vi "test_scd_main.vi"(8 "error in":errorcluster) -> (0 "error out":errorcluster)   [LabVIEW 2023, in "horiba.test.lvlib"]
uses:
  horiba.test.lvlib
  Classes/SCD/SCD.lvclass
  <vilib>/addons/_JKI Toolkits/Caraya/classes/Test/Test.lvclass
  C:/Projects/Horiba/horiba-labview-sdk/Source/Classes/GenericDevice/GenericDevice.lvclass
  C:/Projects/Horiba/horiba-labview-sdk/Source/Classes/SCD/SCD.lvclass
panel:
  # "Connector Pane"
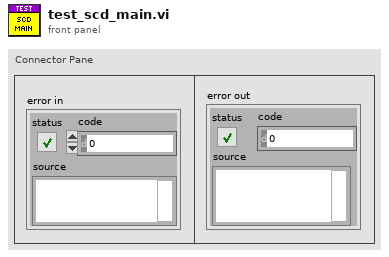
[diagram p1: front panel]
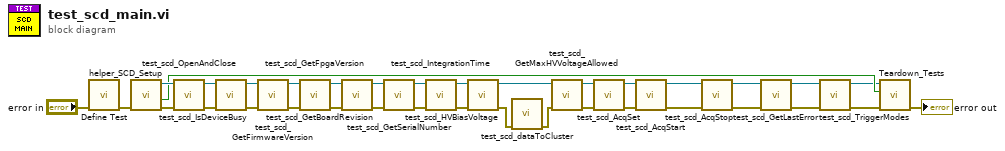
[diagram p0: block diagram]
diagram:
  n1 = call <vilib>:"Define Test.vi"("error in (no error)"="error in") -> ("error out"=w35:errorcluster)  [unwired: 9 in, 1 out]
  n2 = call "helper_SCD_Setup.vi"("error in"=w35) -> ("error out"=w33:errorcluster, "Module Was Already Running?"=w27:bool, "SCD out"=w34:refnum<class "SCD.lvclass">)  [unwired: 7 in, 1 out]
  n3 = call "test_scd_OpenAndClose.vi"("error in"=w33, "SCD in"=w34) -> ("error out"=w31:errorcluster, "SCD out"=w32:refnum<class "SCD.lvclass">)  [unwired: 8 in]
  n4 = call "test_scd_IsDeviceBusy.vi"("error in"=w31, "SCD in"=w32) -> ("error out"=w29:errorcluster, "SCD out"=w30:refnum<class "SCD.lvclass">)  [unwired: 8 in]
  n5 = call "test_scd_GetFirmwareVersion.vi"("error in"=w29, "SCD in"=w30) -> ("error out"=w28:errorcluster, "SCD out"=w25:refnum<class "SCD.lvclass">)  [unwired: 8 in]
  n6 = call "test_scd_GetFpgaVersion.vi"("error in"=w28, "SCD in"=w25) -> ("error out"=w26:errorcluster, "SCD out"=w23:refnum<class "SCD.lvclass">)  [unwired: 8 in]
  n7 = call "test_scd_GetBoardRevision.vi"("error in"=w26, "SCD in"=w23) -> ("error out"=w24:errorcluster, "SCD out"=w21:refnum<class "SCD.lvclass">)  [unwired: 8 in]
  n8 = call "test_scd_GetSerialNumber.vi"("error in"=w24, "SCD in"=w21) -> ("error out"=w22:errorcluster, "SCD out"=w19:refnum<class "SCD.lvclass">)  [unwired: 8 in]
  n9 = call "test_scd_IntegrationTime.vi"("error in"=w22, "SCD in"=w19) -> ("error out"=w20:errorcluster, "SCD out"=w17:refnum<class "SCD.lvclass">)  [unwired: 8 in]
  n10 = call "test_scd_HVBiasVoltage.vi"("error in"=w20, "SCD in"=w17) -> ("error out"=w18:errorcluster, "SCD out"=w8:refnum<class "SCD.lvclass">)  [unwired: 8 in]
  n11 = call "test_scd_dataToCluster.vi"("error in (no error)"=w18) -> ("error out"=w11:errorcluster)  [unwired: 10 in]
  n12 = call "test_scd_GetMaxHVVoltageAllowed.vi"("error in"=w11, "SCD in"=w8) -> ("error out"=w16:errorcluster, "SCD out"=w14:refnum<class "SCD.lvclass">)  [unwired: 8 in]
  n13 = call "test_scd_AcqSet.vi"("error in"=w16, "SCD in"=w14) -> ("error out"=w15:errorcluster, "SCD out"=w9:refnum<class "SCD.lvclass">)  [unwired: 8 in]
  n14 = call "test_scd_AcqStart.vi"("error in"=w15, "SCD in"=w9) -> ("error out"=w10:errorcluster, "SCD out"=w4:refnum<class "SCD.lvclass">)  [unwired: 8 in]
  n15 = call "test_scd_AcqStop.vi"("error in"=w10, "SCD in"=w4) -> ("error out"=w5:errorcluster, "SCD out"=w2:refnum<class "SCD.lvclass">)  [unwired: 8 in]
  n16 = call "test_scd_GetLastError.vi"("error in"=w5, "SCD in"=w2) -> ("error out"=w3:errorcluster, "SCD out"=w1:refnum<class "SCD.lvclass">)  [unwired: 8 in]
  n17 = call "test_scd_TriggerModes.vi"("error in"=w3, "SCD in"=w1) -> ("error out"=w7:errorcluster, "SCD out"=w6:refnum<class "SCD.lvclass">)  [unwired: 8 in]
  n18 = call "Teardown_Tests.vi"("error in"=w7, "Module Was Already Running?"=w27, "horiba.lvlib:GenericDevice"=w6) -> ("error out"=→"error out":errorcluster)  [unwired: 7 in, 1 out]
